vi "Capture Example.vi"() -> ()   [LabVIEW 2020]
uses:
  g_ar_toolkit.capture/CameraStream/CameraStream.lvclass/CameraStream.ctl
  g_ar_toolkit.image/CreateEmptyImageARGB.vi
  g_ar_toolkit.image/DrawImageToPictureARGB.vi
  g_ar_toolkit.image/CreateEmptyImageARGB.vi/3321fa97-f432-4e1e-8db9-a0df79aed21b.vi
  g_ar_toolkit.image/DrawImageToPictureARGB.vi/8cd07b1b-062e-4fe4-9e87-2eb3dc89fe0e.vi
  g_ar_toolkit.image/ARGBColourToU32.vi
  <vilib>/Utility/error.llb/Error Cluster From Error Code.vi
  g_ar_toolkit.capture/CameraStream/CameraStream.lvclass
  g_ar_toolkit.capture/CameraManager/CameraManager.lvclass
  g_ar_toolkit.image/g_ar_toolkit.image.lvlib
panel:
  in  "Start/Stop":bool
  in  "Format":string(combo)
  in  "Source":string(combo)
  in  "Enumerate":bool
  in  "Erase":bool
  in  "Picture Zoom":dbl=1.0 min=0.0001 max=10.0 step=0.1
  out "2D Picture":picture
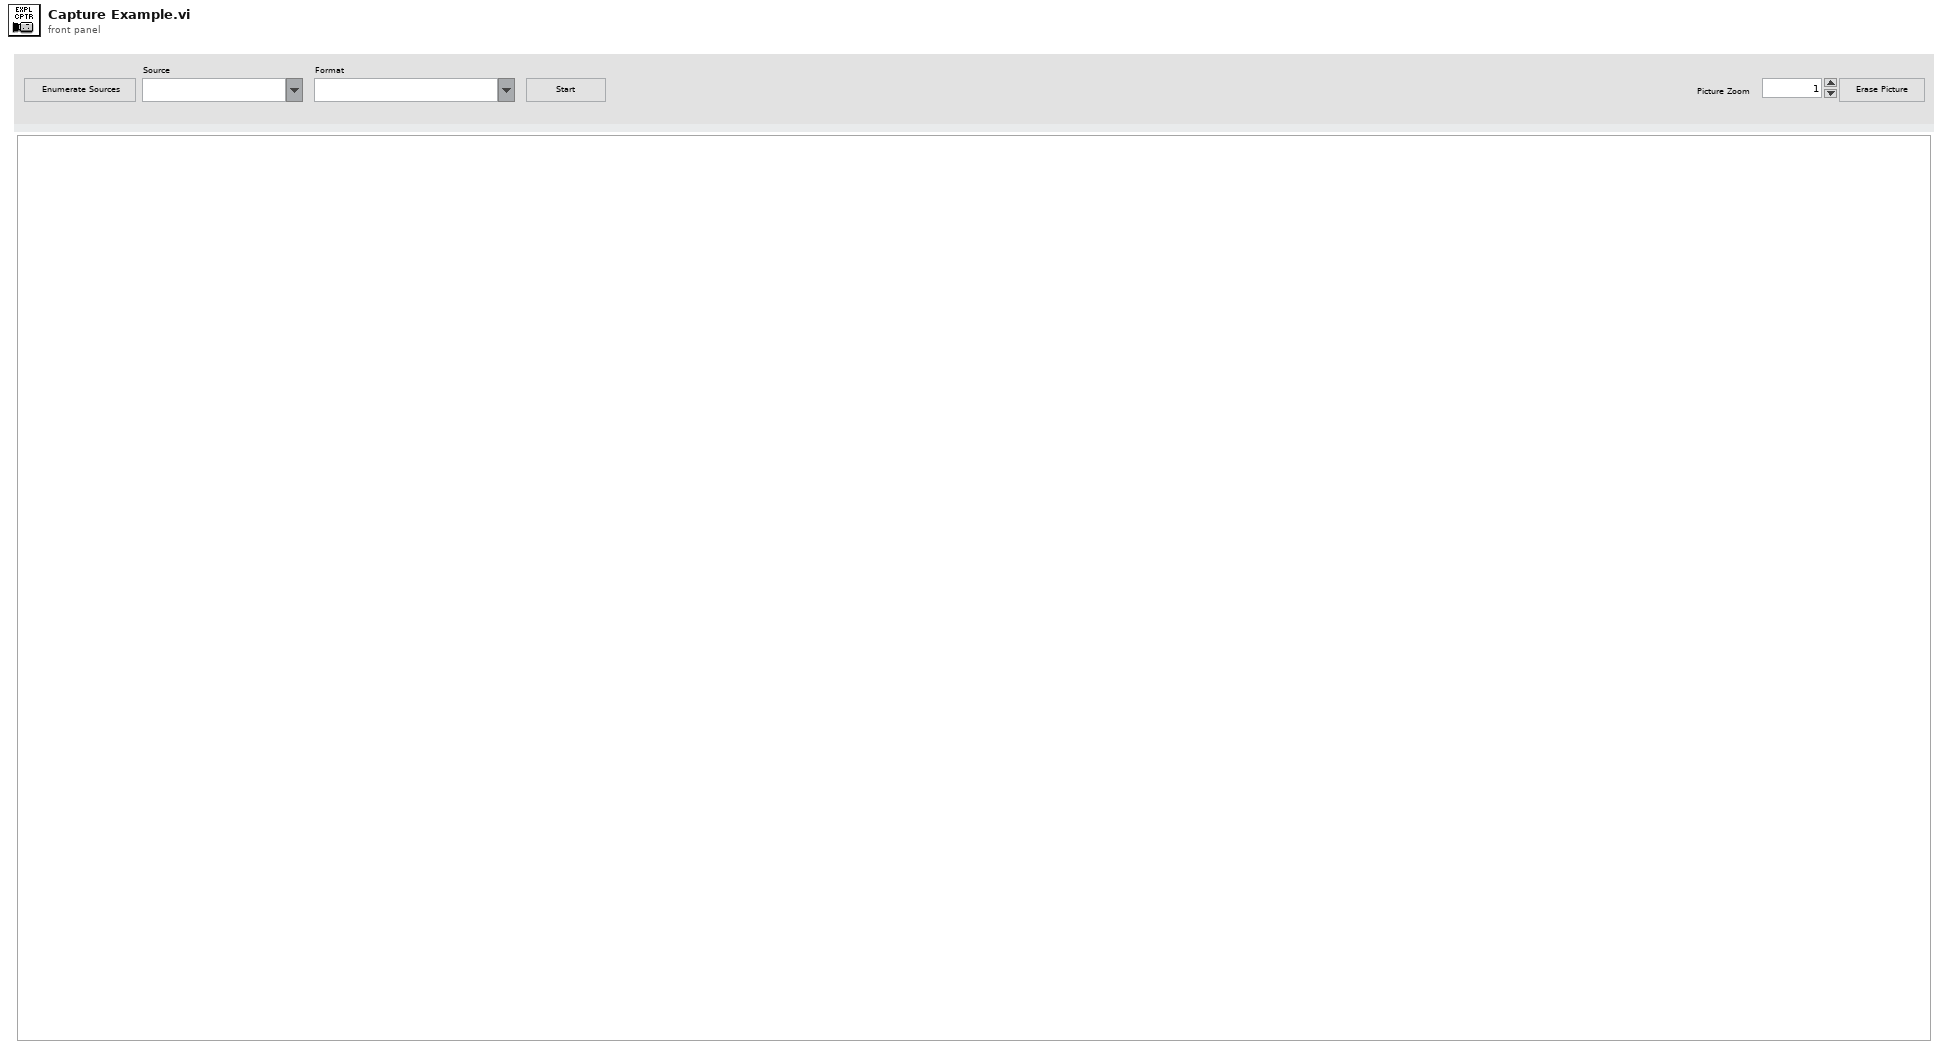
[diagram p1: front panel]
types:
  T1 = enum8{"Enabled", "Disabled", "Disabled and Grayed Out"}
  T2 = typedef "g_ar_toolkit.capture.lvlib/CameraManager.lvclass/Device Enumeration.ctl" = cluster{"Name":string, "Streams":set{T3}}
  T3 = typedef "g_ar_toolkit.capture.lvlib/CameraManager.lvclass/Stream Parameters.ctl" = cluster{"Width":u16, "Height":u16, "FPS":u8}
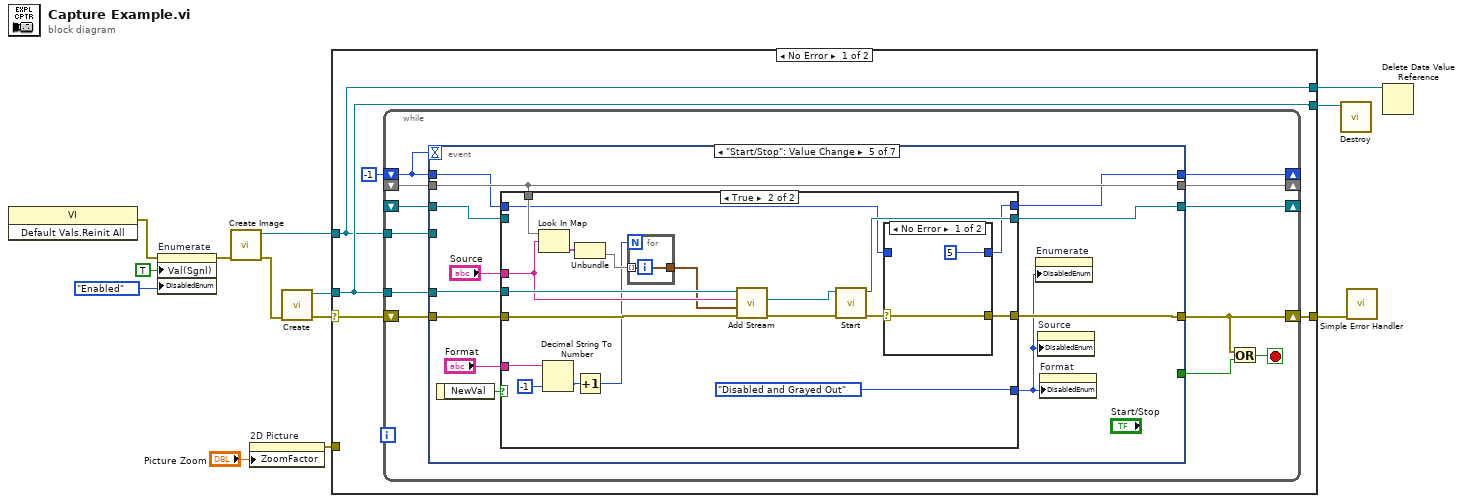
[diagram p0: block diagram]
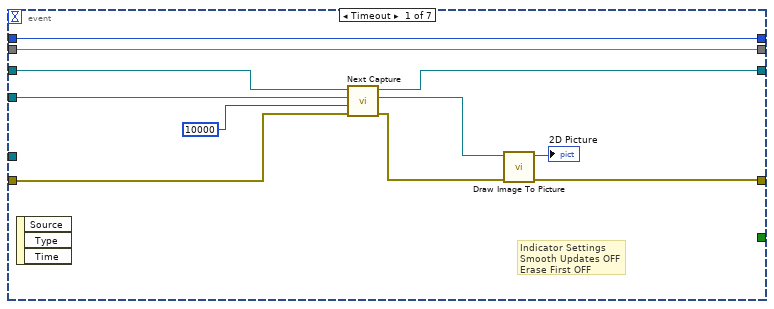
[diagram p2: hidden frame]
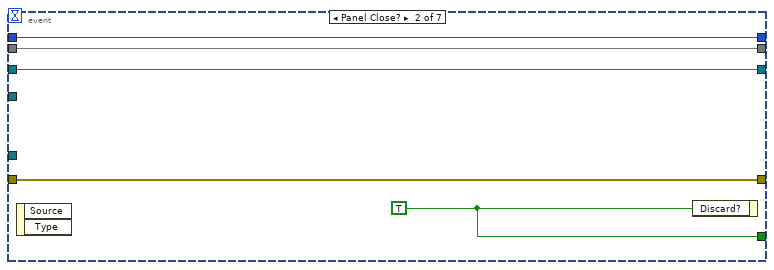
[diagram p3: hidden frame]
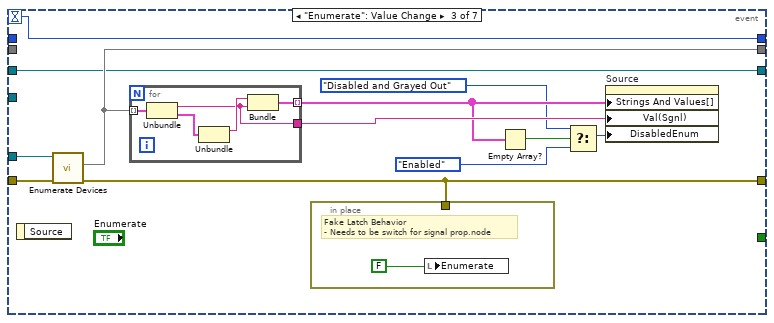
[diagram p4: hidden frame]
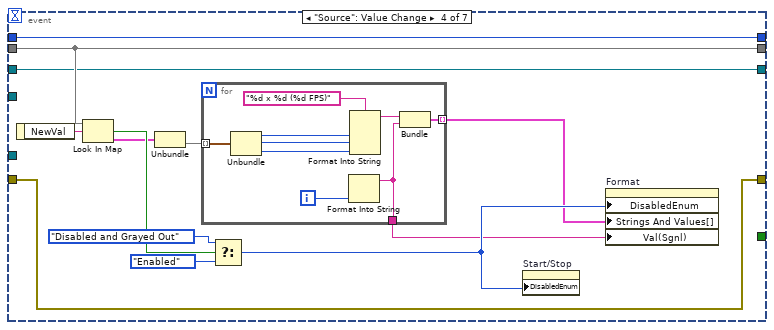
[diagram p5: hidden frame]
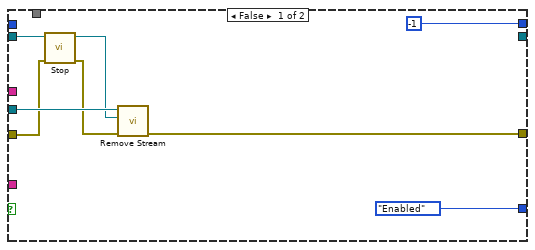
[diagram p6: hidden frame]
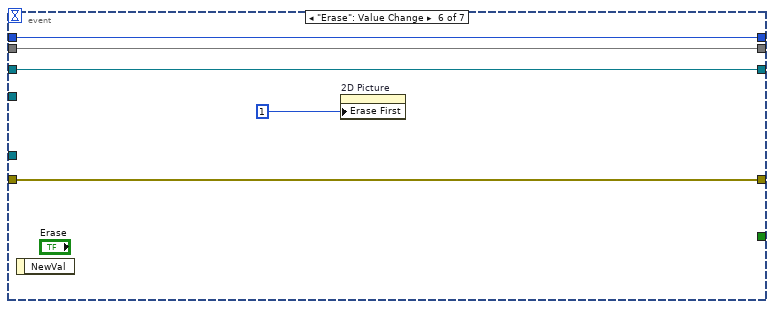
[diagram p8: hidden frame]
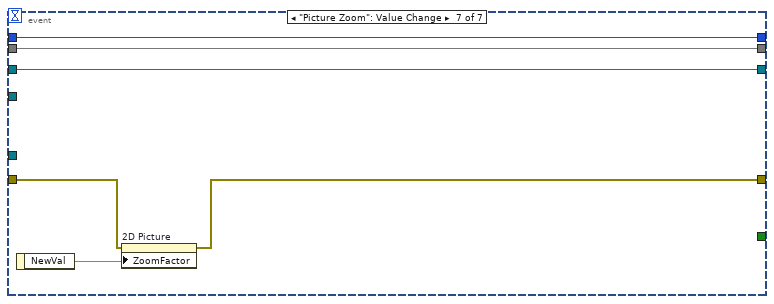
[diagram p9: hidden frame]
diagram:
  n1 = invoke class="VI" method="Default Vals.Reinit All"() -> (error out=w5:errorcluster)  [unwired: 3 in, 2 out]
  n2 = property on="Enumerate" class="Bool (strict)"(error in=w5, "Val(Sgnl)"=TRUE ("Value (Signaling)"), "DisabledEnum"=T1."Enabled" ("Disabled")) -> (error out=w1:errorcluster)  [unwired: 1 in, 1 out]
  n3 = call-poly "Create Image.vi"("error in (no error)"=w1) -> ("error out"=w4:errorcluster, "New ARGB Image"=w10:refnum<data-value>)  [unwired: 9 in]
  n4 = property on="2D Picture" class="Pict"("ZoomFactor"="Picture Zoom") -> (error out=w9:errorcluster)  [unwired: 2 in, 1 out]
  n5 = call "Create.vi"("error in (no error)"=w4) -> ("error out"=w13:errorcluster, "CameraManager"=w2:refnum<data-value>)  [unwired: 9 in]
  n6 = case shown="No Error" w13 {
    selector: w13 -> [w18 w142]
    tunnel: w2 -> [w17 w144]
    tunnel: [w17 w144] -> w12
    tunnel: w10 -> [w15 w143]
    tunnel: w9 -> [_ _]
    tunnel: [w15 w143] -> w7
    tunnel: [w14 w142] -> w6
    frame No Error {
      n7 = while {
        tunnel: w17 -> [w30]
        shift-right: [w28] -> _
        shift-left: _ -> [w27]
        shift-right: [w26] -> w14
        shift-left: w18 -> [w29]
        shift-right: [w23] -> _
        shift-left: -1 -> [w22]
        shift-right: [w21] -> _
        shift-left: _ -> [w20]
        tunnel: w15 -> [w19]
        stop <- w25 stop-if-true
        n8 = event shown="[4] \"Start/Stop\": Value Change" {
          selector: _ -> [_ _ _ _ _ _ _]
          dyn-events: _ -> [_ _ _ _ _ _ _]
          timeout: w22 -> [_ _ w53 _ _ _ _]
          tunnel: w30 -> [_ _ w58 _ w94 _ _]
          tunnel: w29 -> [w33 w45 w57 w65 w95 w132 w138]
          tunnel: [w41 w44 w56 w77 w93 w135 w136] -> w28
          tunnel: w27 -> [w41 w44 _ w77 w93 w135 w136]
          tunnel: [w32 w45 w54 w65 w92 w132 w137] -> w26
          tunnel: [_ w46 _ _ _ _ _] -> w24
          tunnel: [w40 w43 w53 w67 w89 w134 w141] -> w23
          tunnel: w22 -> [w40 w43 _ w67 w90 w134 w141]
          tunnel: [w38 w42 w52 w66 w91 w133 w140] -> w21
          tunnel: w20 -> [w39 w42 w52 w66 w88 w133 w140]
          tunnel: w19 -> [w37 _ _ _ _ _ _]
          event Timeout {
            # "Indicator Settings\nSmooth Updates OFF\nErase First OFF"
            n9 = event-data() -> ()  [unwired: 1 in, 3 out]
            n10 = call "Next Capture.vi"("error in (no error)"=w33, "timeout (ms)"=u16 10000, "ARGB Image Destination"=w37, "Stream"=w39) -> ("error out"=w34:errorcluster, "ARGB Image (duplicate)"=w35:refnum<data-value>, "Stream (duplicate)"=w38:refnum<data-value>)  [unwired: 5 in]
            n11 = call-poly "Draw Image To Picture.vi"("error in (no error)"=w34, "ARGB Image Source"=w35) -> ("error out"=w32:errorcluster, "Picture"=→"2D Picture":picture)  [unwired: 8 in]
          }
          event Panel Close? {
            w46 = TRUE ("Discard?")
            n12 = event-data() -> ()  [unwired: 1 in, 2 out]
            n13 = event-data("Discard?"=w46) -> ()  [unwired: 1 in, 1 out]
          }
          event "Enumerate": Value Change {
            n14 = event-data() -> ()  [unwired: 1 in, 1 out]
            n15 = call "Enumerate Devices.vi"("error in (no error)"=w57, "CameraManager"=w58) -> ("error out"=w54:errorcluster, "Devices"=w56:map{string, T2})  [unwired: 7 in, 1 out]
            n16 = for {
              tunnel: w56 -> [w64] mode=indexing
              tunnel: [w61] -> w50 mode=indexing
              tunnel: [w60] -> w55
              n17 = Unbundle(w64) -> ("id"=w60:string, "Info"=w63:T2)
              n18 = Unbundle(w63) -> ("Name"=w62:string)  [unwired: 1 out]
              n19 = Bundle("Name"=w62, "id"=w60) -> (w61:cluster{"Name":string, "id":string})  [unwired: 1 in]
            }
            n20 = in-place {
              in-place-border: w54 -> [_]
              # "Fake Latch Behavior\n- Needs to be switch for signal prop.node"
              n21 = local write "Enumerate"(FALSE ("Re-Enumerate Sources")) -> ()
            }
            n22 = Empty Array?(array=w50) -> (empty?=w51:bool)
            n23 = Select(t=T1."Disabled and Grayed Out", s=w51, f=T1."Enabled" ("Disabled")) -> (s? t:f=w47:T1)
            n24 = property on="Source" class="CmbBox"("Strings And Values[]"=w50, "Val(Sgnl)"=w55, "DisabledEnum"=w47) -> ()  [unwired: 2 in, 2 out]
          }
          event "Source": Value Change {
            n25 = event-data() -> ("NewVal"=w76:string)  [unwired: 1 in]
            n26 = Look In Map(map=w77, key=w76) -> (key not found?=w75:bool, value=w72:T2)  [unwired: 1 in]
            n27 = Unbundle(w72) -> ("Streams"=w71:set{T3})  [unwired: 1 out]
            n28 = for {
              tunnel: w71 -> [w81] mode=indexing
              tunnel: [w84] -> w69 mode=indexing
              tunnel: [w83] -> w68
              i -> [w86]
              n29 = Unbundle(w81) -> ("Width"=w80:u16, "Height"=w79:u16, "FPS"=w78:u8)
              n30 = Format Into String(w86) -> (resulting string=w83:string)  [unwired: 3 in, 1 out]
              n31 = Format Into String(format string="%d x %d (%d FPS)", w80, w79, w78) -> (resulting string=w85:string)  [unwired: 2 in, 1 out]
              n32 = Bundle(w85, w83) -> (w84:cluster{string, string})  [unwired: 1 in]
            }
            n33 = Select(t=T1."Disabled and Grayed Out" ("Disabled"), s=w75, f=T1."Enabled") -> (s? t:f=w70:T1)
            n34 = property on="Start/Stop" class="Bool (strict)"("DisabledEnum"=w70) -> ()  [unwired: 2 in, 2 out]
            n35 = property on="Format" class="CmbBox"("DisabledEnum"=w70, "Strings And Values[]"=w69, "Val(Sgnl)"=w68) -> ()  [unwired: 2 in, 2 out]
          }
          event "Start/Stop": Value Change {
            n36 = event-data() -> ("NewVal"=w98:bool)  [unwired: 1 in]
            n37 = case shown="True" w98 {
              tunnel: "Source" -> [_ w121]
              tunnel: "Format" -> [_ w120]
              tunnel: w95 -> [w103 w124]
              tunnel: w94 -> [w105 w125]
              tunnel: w93 -> [_ w123]
              tunnel: [w100 w115] -> w92
              tunnel: [_ w113] -> w91
              tunnel: w90 -> [_ w112]
              tunnel: [-1 w111] -> w89
              tunnel: w88 -> [w106 _]
              tunnel: [T1."Enabled" ("Disabled") T1."Disabled and Grayed Out" ("Disabled")] -> w87
              frame False {
                n38 = call "Stop.vi"("error in (no error)"=w103, "Stream"=w106) -> ("error out"=w102:errorcluster, "Stream (duplicate)"=w104:refnum<data-value>)  [unwired: 8 in]
                n39 = call "Remove Stream.vi"("error in (no error)"=w102, "Stream"=w104, "CameraManager"=w105) -> ("error out"=w100:errorcluster)  [unwired: 7 in, 1 out]
              }
              frame True {
                n40 = Look In Map(map=w123, key=w121) -> (value=w122:T2)  [unwired: 1 in, 1 out]
                n41 = Decimal String To Number(string=w120, default (0L)=-1 ("default (0 I32)")) -> (number=w116:i32)  [unwired: 1 in, 1 out]
                n42 = Unbundle(w122) -> ("Streams"=w119:set{T3})  [unwired: 1 out]
                n43 = Increment(x=w116) -> (x+1=w117:i32)
                n44 = for {
                  N: w117 -> [_]
                  tunnel: w119 -> [w130] mode=indexing
                  tunnel: [w130] -> w107
                }
                n45 = call "Add Stream.vi"("error in (no error)"=w124, "Desired Stream Parameters"=w107, "Device ID"=w121, "CameraManager"=w125) -> ("error out"=w109:errorcluster, "Stream"=w110:refnum<data-value>)  [unwired: 5 in, 1 out]
                n46 = call "Start.vi"("error in (no error)"=w109, "Stream"=w110) -> ("error out"=w114:errorcluster, "Stream (duplicate)"=w113:refnum<data-value>)  [unwired: 8 in]
                n47 = case shown="No Error" w114 {
                  selector: w114 -> [w127 w128]
                  tunnel: [w127 w128] -> w115
                  tunnel: w112 -> [_ w129]
                  tunnel: [5 w129] -> w111
                  frame No Error {
                  }
                  frame Error {
                  }
                }
              }
            }
            n48 = property on="Enumerate" class="Bool (strict)"("DisabledEnum"=w87) -> ()  [unwired: 2 in, 2 out]
            n49 = property on="Source" class="CmbBox"("DisabledEnum"=w87) -> ()  [unwired: 2 in, 2 out]
            n50 = property on="Format" class="CmbBox"("DisabledEnum"=w87) -> ()  [unwired: 2 in, 2 out]
          }
          event "Erase": Value Change {
            n51 = event-data() -> ()  [unwired: 1 in, 1 out]
            n52 = property on="2D Picture" class="Pict"("Erase First"=u8 1) -> ()  [unwired: 2 in, 2 out]
          }
          event "Picture Zoom": Value Change {
            n53 = event-data() -> ("NewVal"=w139:dbl)  [unwired: 1 in]
            n54 = property on="2D Picture" class="Pict"(error in=w138, "ZoomFactor"=w139) -> (error out=w137:errorcluster)  [unwired: 1 in, 1 out]
          }
        }
        n55 = Or(x=w26, y=w24) -> (x .or. y?=w25:bool)
      }
    }
    frame Error {
    }
  }
  n56 = call "Destroy.vi"("CameraManager"=w12) -> ()  [unwired: 10 in, 1 out]
  n57 = call <vilib>:"Simple Error Handler.vi"("error in (no error)"=w6) -> ()  [unwired: 4 in, 5 out]
  n58 = Delete Data Value Reference(data value reference=w7) -> ()  [unwired: 1 in, 2 out]
